vi "Configure Waveform Modifier.vi"(5 "Waveform Modifier (0: Noise)":u16(ring) items=["Noise", "External Signal", "Both"], 6 "Noise Level (10 %)":dbl=10.0 min=0.0 max=50.0 format="%#.6g", 7 "Enable Waveform Modifier (T: Enable)":bool=TRUE, 8 "error in (no error)":errorcluster, 10 "Channel (0: Channel 1)":T1 items=["Channel 1", "Channel 2"], 11 "VISA resource name":refnum<visa-resource-name>) -> (0 "error out":errorcluster, 3 "VISA resource name out":refnum<visa-resource-name>)   [LabVIEW 2009, in "Tektronix AFG 3000 Series.lvlib"]
doc: "Configures whether the function generator adds internal noise, external signal or both to a specified channel."
uses:
  Tektronix AFG 3000 Series.lvlib
  controls.llb/Channel.ctl
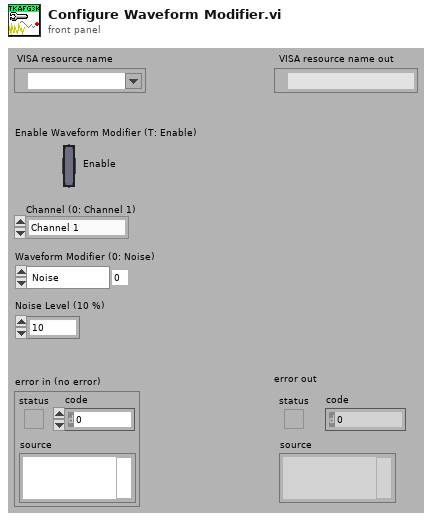
[diagram p1: front panel]
types:
  T1 = typedef "Channel.ctl" = u16
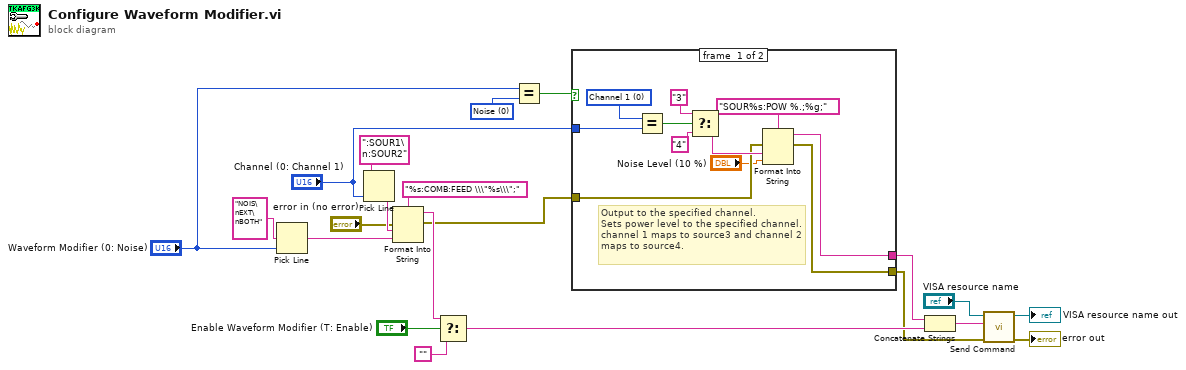
[diagram p0: block diagram]
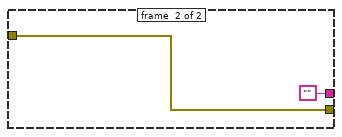
[diagram p2: hidden frame]
diagram:
  w12 = u16 0 items=["Noise", "Signal", "Both"] ("Appendant (0: Noise)")
  n1 = Pick Line(multi-line string="NOIS\nEXT\nBOTH", line index="Waveform Modifier (0: Noise)") -> (output string=w16:string)  [unwired: 1 out]
  n2 = Pick Line(multi-line string=":SOUR1\n:SOUR2" ("string (\"\")"), line index="Channel (0: Channel 1)") -> (output string=w15:string)  [unwired: 1 out]
  n3 = Format Into String(format string="%s:COMB:FEED \\\"%s\\\";", error in="error in (no error)", w15, w16) -> (resulting string=w14:string, error out=w2:errorcluster)  [unwired: 1 in]
  n4 = Select(t=w14, s="Enable Waveform Modifier (T: Enable)", f="") -> (s? t:f=w7:string)
  n5 = Equal?(x="Waveform Modifier (0: Noise)", y=w12) -> (x = y?=w11:bool)
  n6 = case shown="True" w11 {
    tunnel: "Channel (0: Channel 1)" -> [w32 _]
    tunnel: w2 -> [w25 w34]
    tunnel: [w22 w34] -> w1
    tunnel: [w23 ""] -> w8
    frame #0 {
      w31 = u16 0 items=["Channel 1", "Channel 2"] ("Channel (0: Channel 1)")
      # "Output to the specified channel. \nSets power level to the specified channel.   \nchannel 1 maps to source3 and channel 2 maps to source4."
      n7 = Equal?(x=w31, y=w32) -> (x = y?=w26:bool)
      n8 = Select(t="3" ("format string"), s=w26, f="4" ("format string")) -> (s? t:f=w28:string)
      n9 = Format Into String(format string="SOUR%s:POW %.;%g;", error in=w25, w28, "Noise Level (10 %)") -> (resulting string=w23:string, error out=w22:errorcluster)  [unwired: 1 in]
    }
    frame #1 {
    }
  }
  n10 = Concatenate Strings(w8, w7) -> (w5:string)
  n11 = call "Send Command.vi"("error in (no error)"=w1, "write buffer"=w5, "VISA resource name"="VISA resource name") -> ("error out"=→"error out":errorcluster, "VISA resource name out"=→"VISA resource name out":refnum<visa-resource-name>)  [unwired: 7 out]
